vi "BRig_RT__Case_Exp__UploadClosedLoop__updateSettings.vi"(9 "input_newSettings":i64[][](array[numeric]), 10 "input_dataLC":u16[](array[numeric]), 11 "input_dataExp":u16[](array[numeric])) -> (2 "output_dataLC":u16[](array[numeric]), 3 "output_dataExp":u16[](array[numeric]))   [LabVIEW 2014]
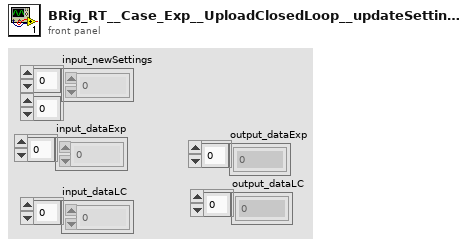
[diagram p1: front panel]
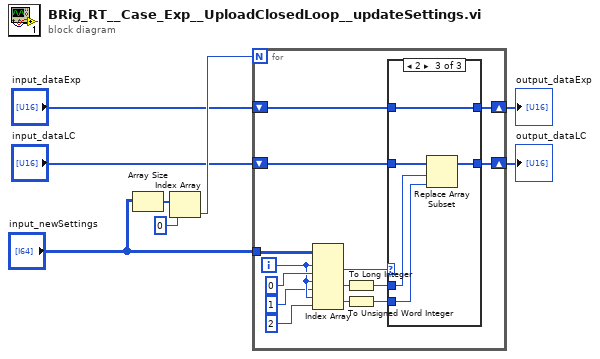
[diagram p0: block diagram]
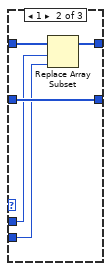
[diagram p3: hidden frame]
diagram:
  n1 = Array Size(array="input_newSettings") -> (size(s)=w8:i32[])
  n2 = Index Array(array=w8, index=0) -> (element=w6:i32)
  n3 = for {
    N: w6 -> [_]
    shift-right: [w17] -> w2
    shift-left: "input_dataExp" -> [w18]
    shift-right: [w16] -> w1
    shift-left: "input_dataLC" -> [w15]
    tunnel: "input_newSettings" -> [w22]
    i -> [w20]
    n4 = Index Array(array=w22, index (row) #1=w20, index (col) #1=0 ("disabled index (col)"), index (row) #2=w20, index (col) #2=1 ("disabled index (col)"), index (row) #3=w20, index (col) #3=2 ("disabled index (col)")) -> (element #1=w19:i64, element #2=w12:i64, element #3=w11:i64)
    n5 = To Long Integer(number=w12) -> (32bit integer=w10:i32)
    n6 = To Unsigned Word Integer(number=w11) -> (unsigned 16bit integer=w9:u16)
    n7 = case shown="2" w19 {
      tunnel: w18 -> [w24 w29 w30]
      tunnel: [w24 w28 w30] -> w17
      tunnel: [w23 w27 w32] -> w16
      tunnel: w15 -> [w23 w27 w31]
      tunnel: w10 -> [_ w26 w34]
      tunnel: w9 -> [_ w25 w33]
      frame 0, Default {
      }
      frame 1 {
        n8 = Replace Array Subset(array=w29, new element=w25, index=w26) -> (w28:u16[])
      }
      frame 2 {
        n9 = Replace Array Subset(array=w31, new element=w33, index=w34) -> (w32:u16[])
      }
    }
  }
  "output_dataExp" <- w2
  "output_dataLC" <- w1
